vi "check syntax.vi"(8 "error in (no error)":errorcluster caption="에러 입력(에러 없음)", 11 "script":string) -> (0 "error out":errorcluster caption="에러 출력", 1 "string error index":cluster{"start":u32, "end":u32}[](array[cluster]), 2 "error":bool, 3 "Script Line 출력":refnum<class "Script Line.lvclass">, 4 "comment exists":bool, 5 "empty script":bool, 6 "comment index":cluster{"start":u32, "end":u32})   [LabVIEW 2020, in "Script Line.lvclass"]
uses:
  Script Line.lvclass
  Controls/function enum.ctl
  Script Line_i2c w/Script Line_i2c w.lvclass
  Script Line_i2c r/Script Line_i2c r.lvclass
  Script Line_i2c sw/Script Line_i2c sw.lvclass
  Script Line_i2c sr/Script Line_i2c sr.lvclass
  Script Line_gpio/Script Line_gpio.lvclass
  Script Line_delay/Script Line_delay.lvclass
  Script Line.lvclass/Script Line.ctl
  Accessors/Write parameter.vi
  Accessors/Write parameter string index.vi
  Accessors/Write script.vi
  Accessors/Read error string index.vi
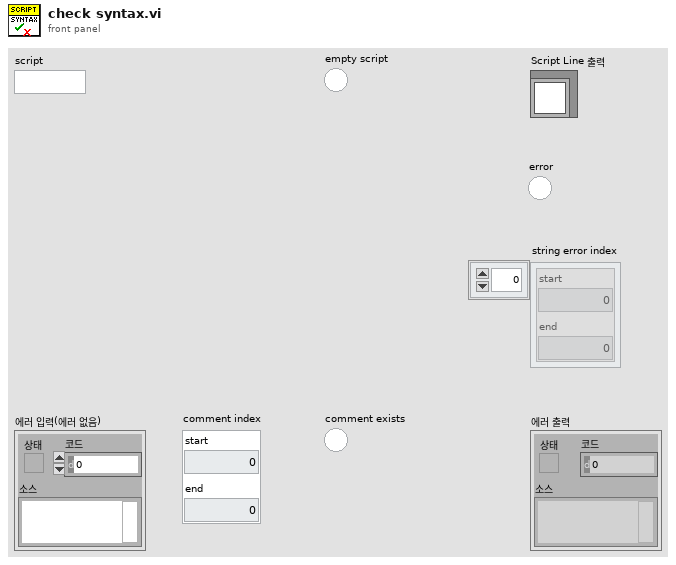
[diagram p1: front panel]
types:
  T1 = typedef "Script Line.lvclass/function enum.ctl" = enum16{"i2c w", "i2c r", "i2c sw", "i2c sr", "gpio", "delay"}
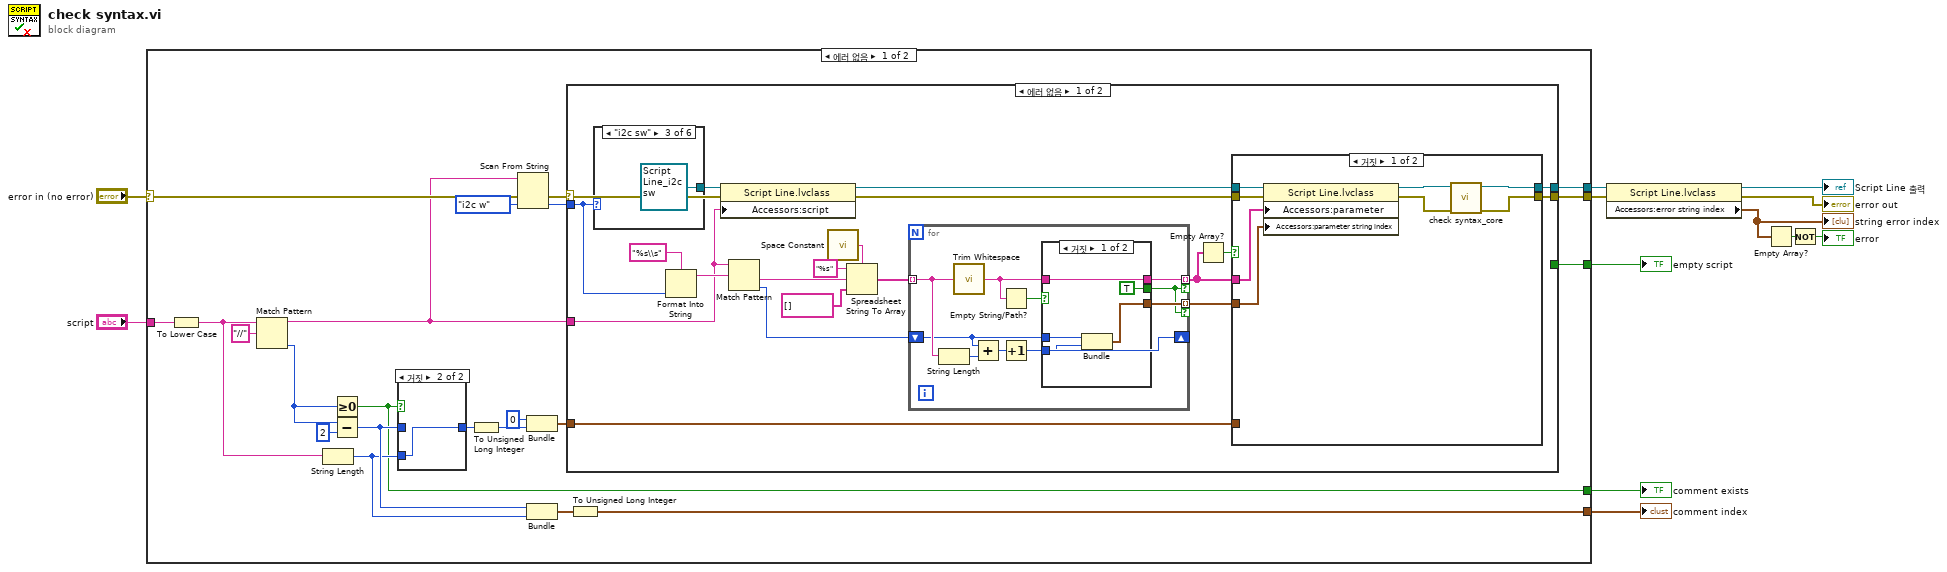
[diagram p0: block diagram]
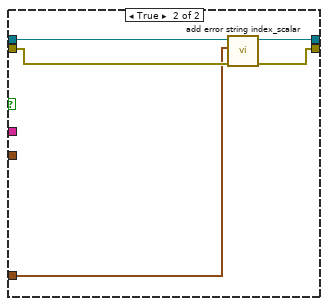
[diagram p3: hidden frame]
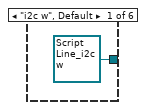
[diagram p5: hidden frame]
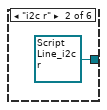
[diagram p6: hidden frame]
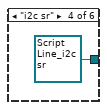
[diagram p7: hidden frame]
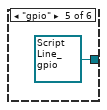
[diagram p8: hidden frame]
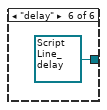
[diagram p9: hidden frame]
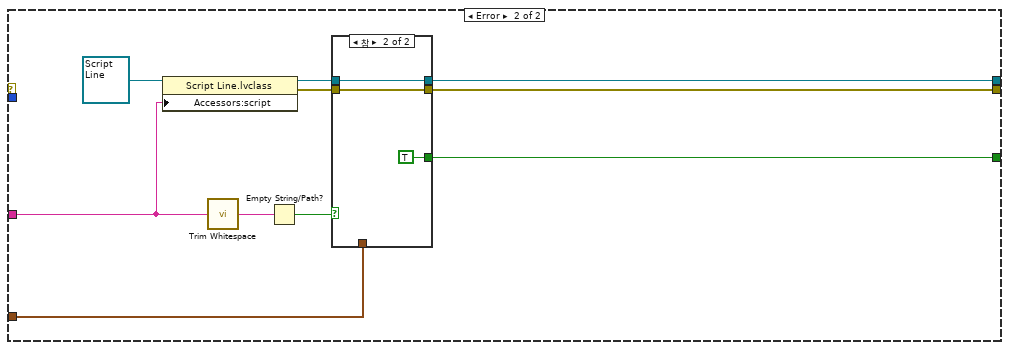
[diagram p10: hidden frame]
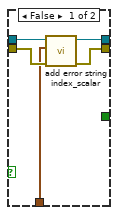
[diagram p11: hidden frame]
diagram:
  n1 = case shown="에러 없음" "error in (no error)" {
    selector: "error in (no error)" -> [w29 w109]
    tunnel: [w31 _] -> w11
    tunnel: "script" -> [w23 _]
    tunnel: [w30 w109] -> w6
    tunnel: [w15 _] -> w3
    tunnel: [w14 _] -> w2
    tunnel: [w13 _] -> w1
    frame No Error {
      n2 = To Lower Case(string=w23) -> (all lower case string=w19:string)
      n3 = Match Pattern(string=w19, regular expression="//" ("정규식")) -> (before substring=w25:string, offset past match=w20:i32)  [unwired: 1 in, 2 out]
      n4 = String Length(string=w19) -> (length=w17:i32)
      n5 = Greater Or Equal To 0?(x=w20) -> (x >= 0?=w14:bool)
      n6 = Subtract(x=w20, y=2) -> (x-y=w18:i32)
      n7 = case shown="거짓" w14 {
        tunnel: [w35 w36] -> w24
        tunnel: w17 -> [_ w36]
        tunnel: w18 -> [w35 _]
        frame True {
        }
        frame False {
        }
      }
      n8 = To Unsigned Long Integer(number=w24) -> (unsigned 32bit integer=w22:u32)
      n9 = Scan From String(input string=w25, error in=w29, default 1=function_enum."i2c w" ("function")) -> (error out=w33:errorcluster, output 1=w32:T1)  [unwired: 2 in, 2 out]
      n10 = Bundle(u32 0, w22) -> (w27:cluster{u32, u32})  [unwired: 1 in]
      n11 = Bundle(w18, w17) -> (w16:cluster{i32, i32})  [unwired: 1 in]
      n12 = case shown="에러 없음" w33 {
        selector: w33 -> [w37 _]
        tunnel: w32 -> [w54 _]
        tunnel: [w43 w98] -> w31
        tunnel: w25 -> [w51 w94]
        tunnel: [w45 w96] -> w30
        tunnel: w27 -> [w39 w95]
        tunnel: [_ w91] -> w13
        frame No Error {
          n13 = case shown="\"i2c sw\"" w54 {
            tunnel: [refnum<class "Script Line_i2c w.lvclass"> refnum ("Script Line_i2c w.lvclass") refnum<class "Script Line_i2c r.lvclass"> refnum ("Script Line_i2c r.lvclass") refnum<class "Script Line_i2c sw.lvclass"> refnum ("Script Line_i2c sw.lvclass") refnum<class "Script Line_i2c sr.lvclass"> refnum ("Script Line_i2c sr.lvclass") refnum<class "Script Line_gpio.lvclass"> refnum ("Script Line_gpio.lvclass") refnum<class "Script Line_delay.lvclass"> refnum ("Script Line_delay.lvclass")] -> w56
            frame "i2c w", Default {
            }
            frame "i2c r" {
            }
            frame "i2c sw" {
            }
            frame "i2c sr" {
            }
            frame "gpio" {
            }
            frame "delay" {
            }
          }
          n14 = Format Into String(format string="%s\\s" ("포맷 문자열"), w54) -> (resulting string=w52:string)  [unwired: 2 in, 1 out]
          n15 = property class="Script Line.lvclass"(reference=w56, error in=w37, "Accessors:script"=w51) -> (reference out=w44:refnum<class "Script Line.lvclass">, error out=w55:errorcluster)
          n16 = Match Pattern(string=w51, regular expression=w52) -> (after substring=w47:string, offset past match=w41:i32)  [unwired: 1 in, 2 out]
          n17 = call <vilib>:"Space Constant.vi"() -> ("String"=w50:string)
          n18 = Spreadsheet String To Array(delimiter (Tab)=w50, format string="%s" ("포맷 문자열"), spreadsheet string=w47, array type (2D Dbl)=string[] []) -> (array=w46:string[])
          n19 = for {
            tunnel: w46 -> [w76] mode=indexing
            tunnel: [w77] -> w40 mode=indexing if=w70
            shift-right: [w72] -> _
            shift-left: w41 -> [w73]
            tunnel: [w71] -> w42 mode=indexing if=w70
            n20 = String Length(string=w76) -> (length=w75:i32)
            n21 = call <vilib>:"Trim Whitespace.vi"("string"=w76) -> ("trimmed string"=w79:string)  [unwired: 1 in]
            n22 = Add(x=w73, y=w75) -> (x+y=w74:i32)
            n23 = Empty String/Path?(string/path=w79) -> (empty?=w78:bool)
            n24 = Increment(x=w74) -> (x+1=w72:i32)
            n25 = case shown="거짓" w78 {
              tunnel: w79 -> [w80 _]
              tunnel: [w80 _] -> w77
              tunnel: [TRUE _] -> w70
              tunnel: w73 -> [w83 _]
              tunnel: w72 -> [w82 _]
              tunnel: [w81 _] -> w71
              frame False {
                n26 = Bundle("offset past match"=w83, w82) -> (w81:cluster{"offset past match":i32, i32})  [unwired: 1 in]
              }
              frame True {
              }
            }
          }
          n27 = Empty Array?(array=w40) -> (empty?=w38:bool)
          n28 = case shown="거짓" w38 {
            tunnel: w55 -> [w64 w67]
            tunnel: [w59 w66] -> w45
            tunnel: w44 -> [w62 w69]
            tunnel: [w57 w68] -> w43
            tunnel: w42 -> [w60 _]
            tunnel: w40 -> [w61 _]
            tunnel: w39 -> [_ w65]
            frame False {
              n29 = property class="Script Line.lvclass"(reference=w62, error in=w64, "Accessors:parameter"=w61, "Accessors:parameter string index"=w60) -> (reference out=w58:refnum<class "Script Line.lvclass">, error out=w63:errorcluster)
              n30 = call-dynamic "check syntax_core.vi"("error in (no error)"=w63, "Script Line 입력"=w58) -> ("error out"=w59:errorcluster, "Script Line 출력"=w57:refnum<class "Script Line.lvclass">)  [unwired: 8 in]
            }
            frame True {
              n31 = call "add error string index_scalar.vi"("error in (no error)"=w67, "index_scalar"=w65, "Script Line 입력"=w69) -> ("error out"=w66:errorcluster, "Script Line 출력"=w68:refnum<class "Script Line.lvclass">)  [unwired: 7 in]
            }
          }
        }
        frame Error {
          n32 = property class="Script Line.lvclass"(reference=refnum<class "Script Line.lvclass"> refnum ("Script Line.lvclass"), "Accessors:script"=w94) -> (reference out=w99:refnum<class "Script Line.lvclass">, error out=w97:errorcluster)  [unwired: 1 in]
          n33 = call <vilib>:"Trim Whitespace.vi"("string"=w94) -> ("trimmed string"=w93:string)  [unwired: 1 in]
          n34 = Empty String/Path?(string/path=w93) -> (empty?=w92:bool)
          n35 = case shown="참" w92 {
            tunnel: w99 -> [w105 w108]
            tunnel: [w104 w108] -> w98
            tunnel: w97 -> [w103 w107]
            tunnel: [w102 w107] -> w96
            tunnel: w95 -> [w101 _]
            tunnel: [_ TRUE] -> w91
            frame False {
              n36 = call "add error string index_scalar.vi"("error in (no error)"=w103, "index_scalar"=w101, "Script Line 입력"=w105) -> ("error out"=w102:errorcluster, "Script Line 출력"=w104:refnum<class "Script Line.lvclass">)  [unwired: 7 in]
            }
            frame True {
            }
          }
        }
      }
      n37 = To Unsigned Long Integer(number=w16) -> (unsigned 32bit integer=w15:cluster{u32, u32})
    }
    frame Error {
    }
  }
  "comment exists" <- w2
  "comment index" <- w3
  "empty script" <- w1
  n38 = property class="Script Line.lvclass"(reference=w11, error in=w6) -> (reference out=→"Script Line 출력":refnum<class "Script Line.lvclass">, error out=→"error out":errorcluster, "Accessors:error string index"=w8:cluster{"start":u32, "end":u32}[])
  "string error index" <- w8
  n39 = Empty Array?(array=w8) -> (empty?=w7:bool)
  n40 = Not(x=w7) -> (.not. x?=→"error":bool)
